vi "Line Detector Create rusin_dat.vi"(6 "New style":bool, 8 "Error In":errorcluster, 9 "header":string, 10 "Fit results":dbl[][](array[numeric]) format="%#_4p", 11 "File Path Control":path) -> (0 "Error Out":errorcluster)   [LabVIEW 2019]
panel:
  # "F0         dF     Ampl   Phase   Xbgrd   Ybgrd"
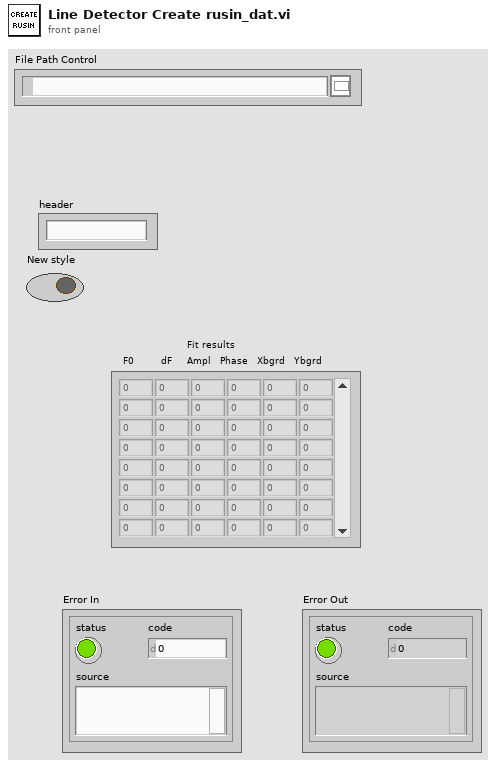
[diagram p1: front panel]
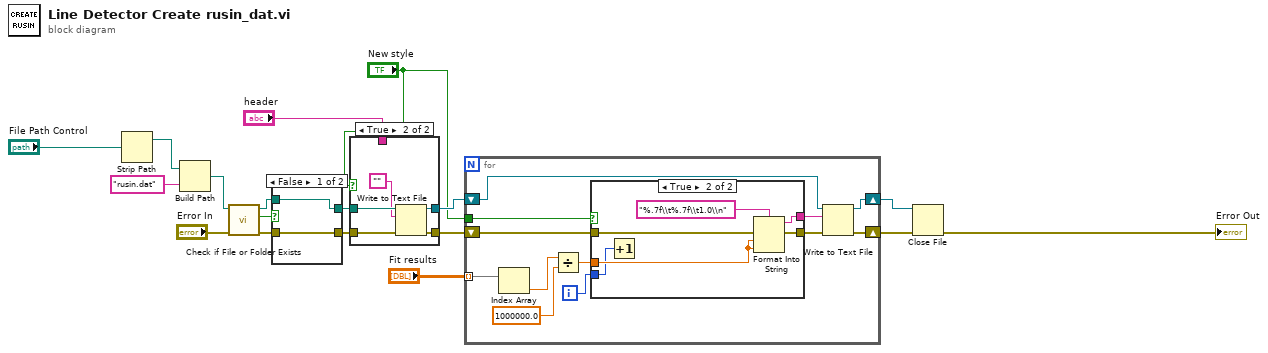
[diagram p0: block diagram]
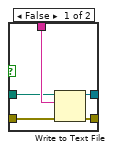
[diagram p2: hidden frame]
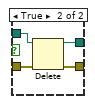
[diagram p3: hidden frame]
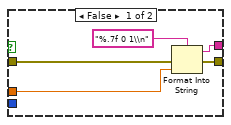
[diagram p4: hidden frame]
diagram:
  n1 = Strip Path(path="File Path Control") -> (stripped path=w17:path)  [unwired: 1 out]
  n2 = Build Path(base path=w17, name or relative path="rusin.dat") -> (appended path=w10:path)
  n3 = call <vilib>:"Check if File or Folder Exists.vi"("error in (no error)"="Error In", "path"=w10) -> ("error out"=w7:errorcluster, "file or folder exists?"=w8:bool, "dup path"=w11:path)  [unwired: 7 in]
  n4 = case shown="False" w8 {
    tunnel: w11 -> [w19 w24]
    tunnel: [w19 w23] -> w9
    tunnel: w7 -> [w20 w22]
    tunnel: [w20 w21] -> w6
    frame False {
    }
    frame True {
      n5 = Delete(path (use dialog)=w24, error in=w22) -> (deleted path=w23:path, error out=w21:errorcluster)  [unwired: 3 in, 1 out]
    }
  }
  n6 = case shown="True" "New style" {
    tunnel: "header" -> [w29 _]
    tunnel: [w28 w34] -> w15
    tunnel: [w27 w33] -> w14
    tunnel: w9 -> [w26 w32]
    tunnel: w6 -> [w25 w31]
    frame False {
      n7 = Write to Text File(file (use dialog)=w26, text=w29, error in=w25) -> (refnum out=w28:refnum<file>, error out=w27:errorcluster)  [unwired: 1 in, 1 out]
    }
    frame True {
      n8 = Write to Text File(file (use dialog)=w32, text="", error in=w31) -> (refnum out=w34:refnum<file>, error out=w33:errorcluster)  [unwired: 1 in, 1 out]
    }
  }
  n9 = for {
    tunnel: "Fit results" -> [w44] mode=indexing
    shift-right: [w38] -> w13
    shift-left: w14 -> [w39]
    shift-right: [w37] -> w12
    shift-left: w15 -> [w46]
    tunnel: "New style" -> [w36]
    i -> [w35]
    n10 = Index Array(array=w44) -> (element=w45:dbl)  [unwired: 1 in]
    n11 = Divide(x=w45, y=1000000.0) -> (x/y=w43:dbl)
    n12 = case shown="True" w36 {
      tunnel: w43 -> [w50 w54]
      tunnel: [w49 w52] -> w41
      tunnel: [w48 w55] -> w40
      tunnel: w39 -> [w47 w56]
      tunnel: w35 -> [_ w53]
      frame False {
        n13 = Format Into String(format string="%.7f 0 1\\n", error in=w47, w50) -> (resulting string=w49:string, error out=w48:errorcluster)  [unwired: 1 in]
      }
      frame True {
        n14 = Increment(x=w53) -> ()  [unwired: 1 out]
        n15 = Format Into String(format string="%.7f\\t%.7f\\t1.0\\n", error in=w56, w54, w54) -> (resulting string=w52:string, error out=w55:errorcluster)  [unwired: 1 in]
      }
    }
    n16 = Write to Text File(file (use dialog)=w46, text=w41, error in=w40) -> (refnum out=w37:refnum<file>, error out=w38:errorcluster)  [unwired: 1 in, 1 out]
  }
  n17 = Close File(refnum=w12, error in=w13) -> (error out=→"Error Out":errorcluster)  [unwired: 1 out]
